vi "cam0#-搜索铜碎-2.vi"(8 "Cut基点":cluster{"X":sgl, "Y":sgl}, 9 "输入参数信息":T5, 11 "images":T4) -> (0 "存在铜碎":bool, 1 "检出点":cluster{"X":sgl, "Y":sgl}[](array[cluster]), 4 "ImageMorphOut":T1)   [LabVIEW 2018]
uses:
  <vilib>/vision/Image Controls.llb/IMAQ Image.ctl
  <vilib>/vision/NI_Vision_Development_Module.lvlib
panel:
  in  "槽口反光排除带区宽度":sgl=25.0
  out "ImageMorphOut 2":T1
  out "错误输出":errorcluster
  out "槽内存在铜碎异常":bool
  out "槽形态断裂情况":i32
  out "槽根部存在铜碎异常":bool
  in  "Keep/Remove Particles (F) 2":bool=TRUE
  in  "Selection Values 2":T3(array[cluster])=[{"Measurement Parameter"=35, "Range Lower Value"=0.0, "Range Upper Value"=50.0, "Range"=FALSE, "Measurement Type"=FALSE}] {"Measurement Parameter" items=["Center of Mass X", "Center of Mass Y", "First Pixel X", "First Pixel Y", "Bounding Rect Left", "Bounding Rect Top", "Bounding Rect Right", "Bounding Rect Bottom", "Max Feret Diameter Start X", "Max Feret Diameter Start Y", "Max Feret Diameter End X", "Max Feret Diameter End Y", "Max Horiz. Segment Length Left", "Max Horiz. Segment Length Right", "Max Horiz. Segment Length Row", "-", "Bounding Rect Width", "Bounding Rect Height", "Bounding Rect Diagonal", "Perimeter", "Convex Hull Perimeter", "Holes' Perimeter", "Max Feret Diameter", "Equivalent Ellipse Major Axis", "Equivalent Ellipse Minor Axis", "Equivalent Ellipse Minor Axis (Feret)", "Equivalent Rect Long Side", "Equivalent Rect Short Side", "Equivalent Rect Diagonal", "Equivalent Rect Short Side (Feret)", "Average Horiz. Segment Length", "Average Vert. Segment Length", "Hydraulic Radius", "Waddel Disk Diameter", "-", "Area", "Holes' Area", "Particle & Holes' Area", "Convex Hull Area", "Image Area", "-", "Number of Holes", "Number of Horiz. Segments", "Number of Vert. Segments", "-", "Orientation", "Max Feret Diameter Orientation", "-", "% Area/Image Area", "% Area/(Particle & Holes' Area)", "Ratio of Equivalent Ellipse Axes", "Ratio of Equivalent Rect Sides", "-", "Elongation Factor", "Compactness Factor", "Heywood Circularity Factor", "Type Factor", "-", "Sum X", "Sum Y", "Sum XX", "Sum XY", "Sum YY", "Sum XXX", "Sum XXY", "Sum XYY", "Sum YYY", "-", "Moment of Inertia XX", "Moment of Inertia XY", "Moment of Inertia YY", "Moment of Inertia XXX", "Moment of Inertia XXY", "Moment of Inertia XYY", "Moment of Inertia YYY", "Norm. Moment of Inertia XX", "Norm. Moment of Inertia XY", "Norm. Moment of Inertia YY", "Norm. Moment of Inertia XXX", "Norm. Moment of Inertia XXY", "Norm. Moment of Inertia XYY", "Norm. Moment of Inertia YYY", "Hu Moment 1", "Hu Moment 2", "Hu Moment 3", "Hu Moment 4", "Hu Moment 5", "Hu Moment 6", "Hu Moment 7"]; "Range Lower Value" format="%.2f"; "Range Upper Value" format="%.2f"}
  out "槽根部断裂型铜碎数量":i32
  in  "Keep/Remove Particles (F)":bool
  in  "Selection Values":T3(array[cluster])=[{"Measurement Parameter"=35, "Range Lower Value"=0.0, "Range Upper Value"=1000.0, "Range"=TRUE, "Measurement Type"=FALSE}] {"Measurement Parameter" items=["Center of Mass X", "Center of Mass Y", "First Pixel X", "First Pixel Y", "Bounding Rect Left", "Bounding Rect Top", "Bounding Rect Right", "Bounding Rect Bottom", "Max Feret Diameter Start X", "Max Feret Diameter Start Y", "Max Feret Diameter End X", "Max Feret Diameter End Y", "Max Horiz. Segment Length Left", "Max Horiz. Segment Length Right", "Max Horiz. Segment Length Row", "-", "Bounding Rect Width", "Bounding Rect Height", "Bounding Rect Diagonal", "Perimeter", "Convex Hull Perimeter", "Holes' Perimeter", "Max Feret Diameter", "Equivalent Ellipse Major Axis", "Equivalent Ellipse Minor Axis", "Equivalent Ellipse Minor Axis (Feret)", "Equivalent Rect Long Side", "Equivalent Rect Short Side", "Equivalent Rect Diagonal", "Equivalent Rect Short Side (Feret)", "Average Horiz. Segment Length", "Average Vert. Segment Length", "Hydraulic Radius", "Waddel Disk Diameter", "-", "Area", "Holes' Area", "Particle & Holes' Area", "Convex Hull Area", "Image Area", "-", "Number of Holes", "Number of Horiz. Segments", "Number of Vert. Segments", "-", "Orientation", "Max Feret Diameter Orientation", "-", "% Area/Image Area", "% Area/(Particle & Holes' Area)", "Ratio of Equivalent Ellipse Axes", "Ratio of Equivalent Rect Sides", "-", "Elongation Factor", "Compactness Factor", "Heywood Circularity Factor", "Type Factor", "-", "Sum X", "Sum Y", "Sum XX", "Sum XY", "Sum YY", "Sum XXX", "Sum XXY", "Sum XYY", "Sum YYY", "-", "Moment of Inertia XX", "Moment of Inertia XY", "Moment of Inertia YY", "Moment of Inertia XXX", "Moment of Inertia XXY", "Moment of Inertia XYY", "Moment of Inertia YYY", "Norm. Moment of Inertia XX", "Norm. Moment of Inertia XY", "Norm. Moment of Inertia YY", "Norm. Moment of Inertia XXX", "Norm. Moment of Inertia XXY", "Norm. Moment of Inertia XYY", "Norm. Moment of Inertia YYY", "Hu Moment 1", "Hu Moment 2", "Hu Moment 3", "Hu Moment 4", "Hu Moment 5", "Hu Moment 6", "Hu Moment 7"]}
  # "180110a-初始版本-测量槽宽"
  # "180126a-将基于边沿检测的铜碎搜索方法改为基于形态学的处理方法"
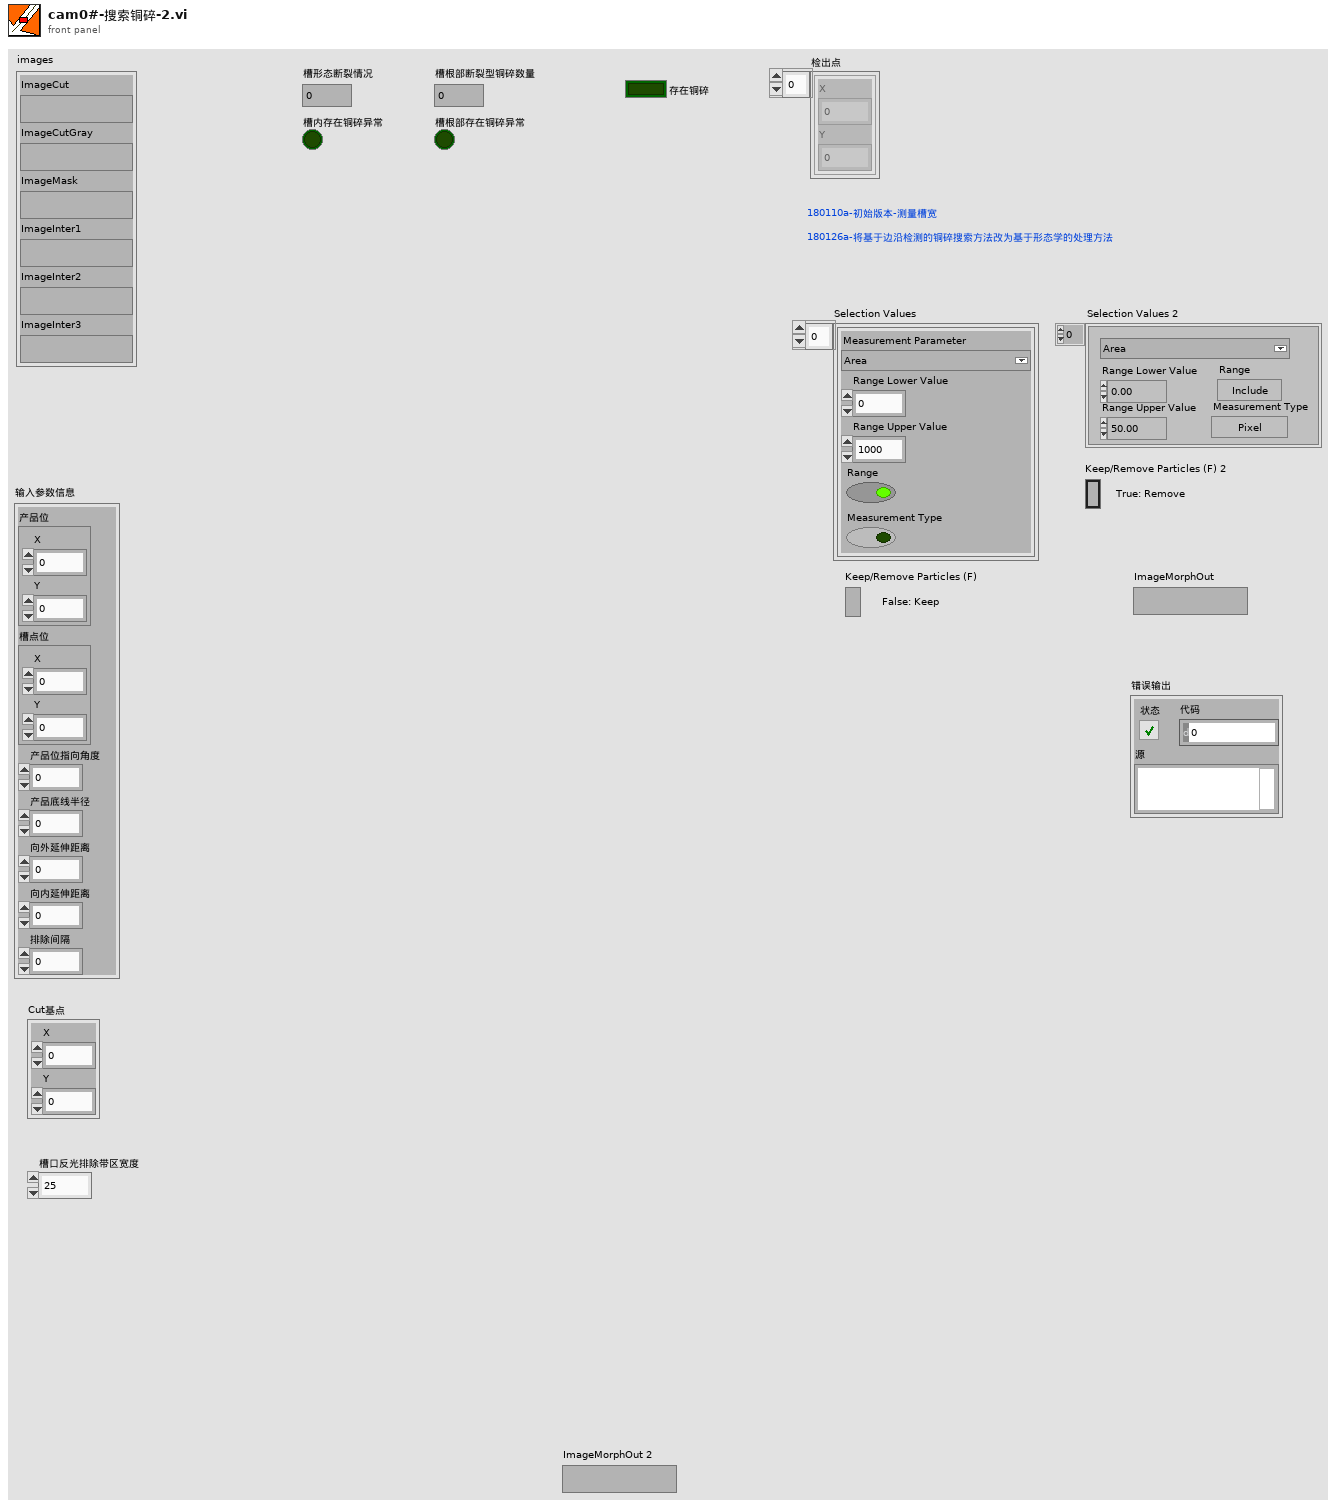
[diagram p1: front panel]
types:
  T1 = typedef "IMAQ Image.ctl" = refnum<image>
  T2 = typedef "Particle Parameters" = i32
  T3 = cluster{"Measurement Parameter":T2, "Range Lower Value":dbl, "Range Upper Value":dbl, "Range":bool, "Measurement Type":bool}[]
  T4 = cluster{"ImageCut":T1, "ImageCutGray":T1, "ImageMask":T1, "ImageInter1":T1, "ImageInter2":T1, "ImageInter3":T1}
  T5 = cluster{"产品位":cluster{"X":sgl, "Y":sgl}, "槽点位":cluster{"X":sgl, "Y":sgl}, "产品位指向角度":sgl, "产品底线半径":sgl, "向外延伸距离":sgl, "向内延伸距离":sgl, "排除间隔":sgl}
  T6 = typedef "IMAQ Circle" = cluster{"Center X":i32, "Center Y":i32, "Inner Radius":i32, "Outer Radius":i32, "Start Angle":dbl, "End Angle":dbl}
  T7 = enum32{"Average", "Min", "Max", "Clear  if < ", "Clear  if < or =", "Clear  if =", "Clear  if > or =", "Clear  if >"}
  T8 = enum32{"AutoM", "Close", "Dilate", "Erode", "Gradient", "Gradient out", "Gradient in", "Hit miss", "Open", "PClose", "POpen", "Thick", "Thin"}
  T9 = typedef "ROI Descriptor" = cluster{"Global Rectangle":i32[], "Contours":cluster{"ID":enum32{"External", "Internal"}, "Type":u32, "Coordinates":i32[]}[]}
  T10 = cluster{"Mean Intensity":sgl, "Standard  Deviation":sgl, "Minimum Intensity":sgl, "Maximum Intensity":sgl}
  T11 = cluster{"Starting Value":sgl, "Interval Width":sgl, "histogram":u32[]}
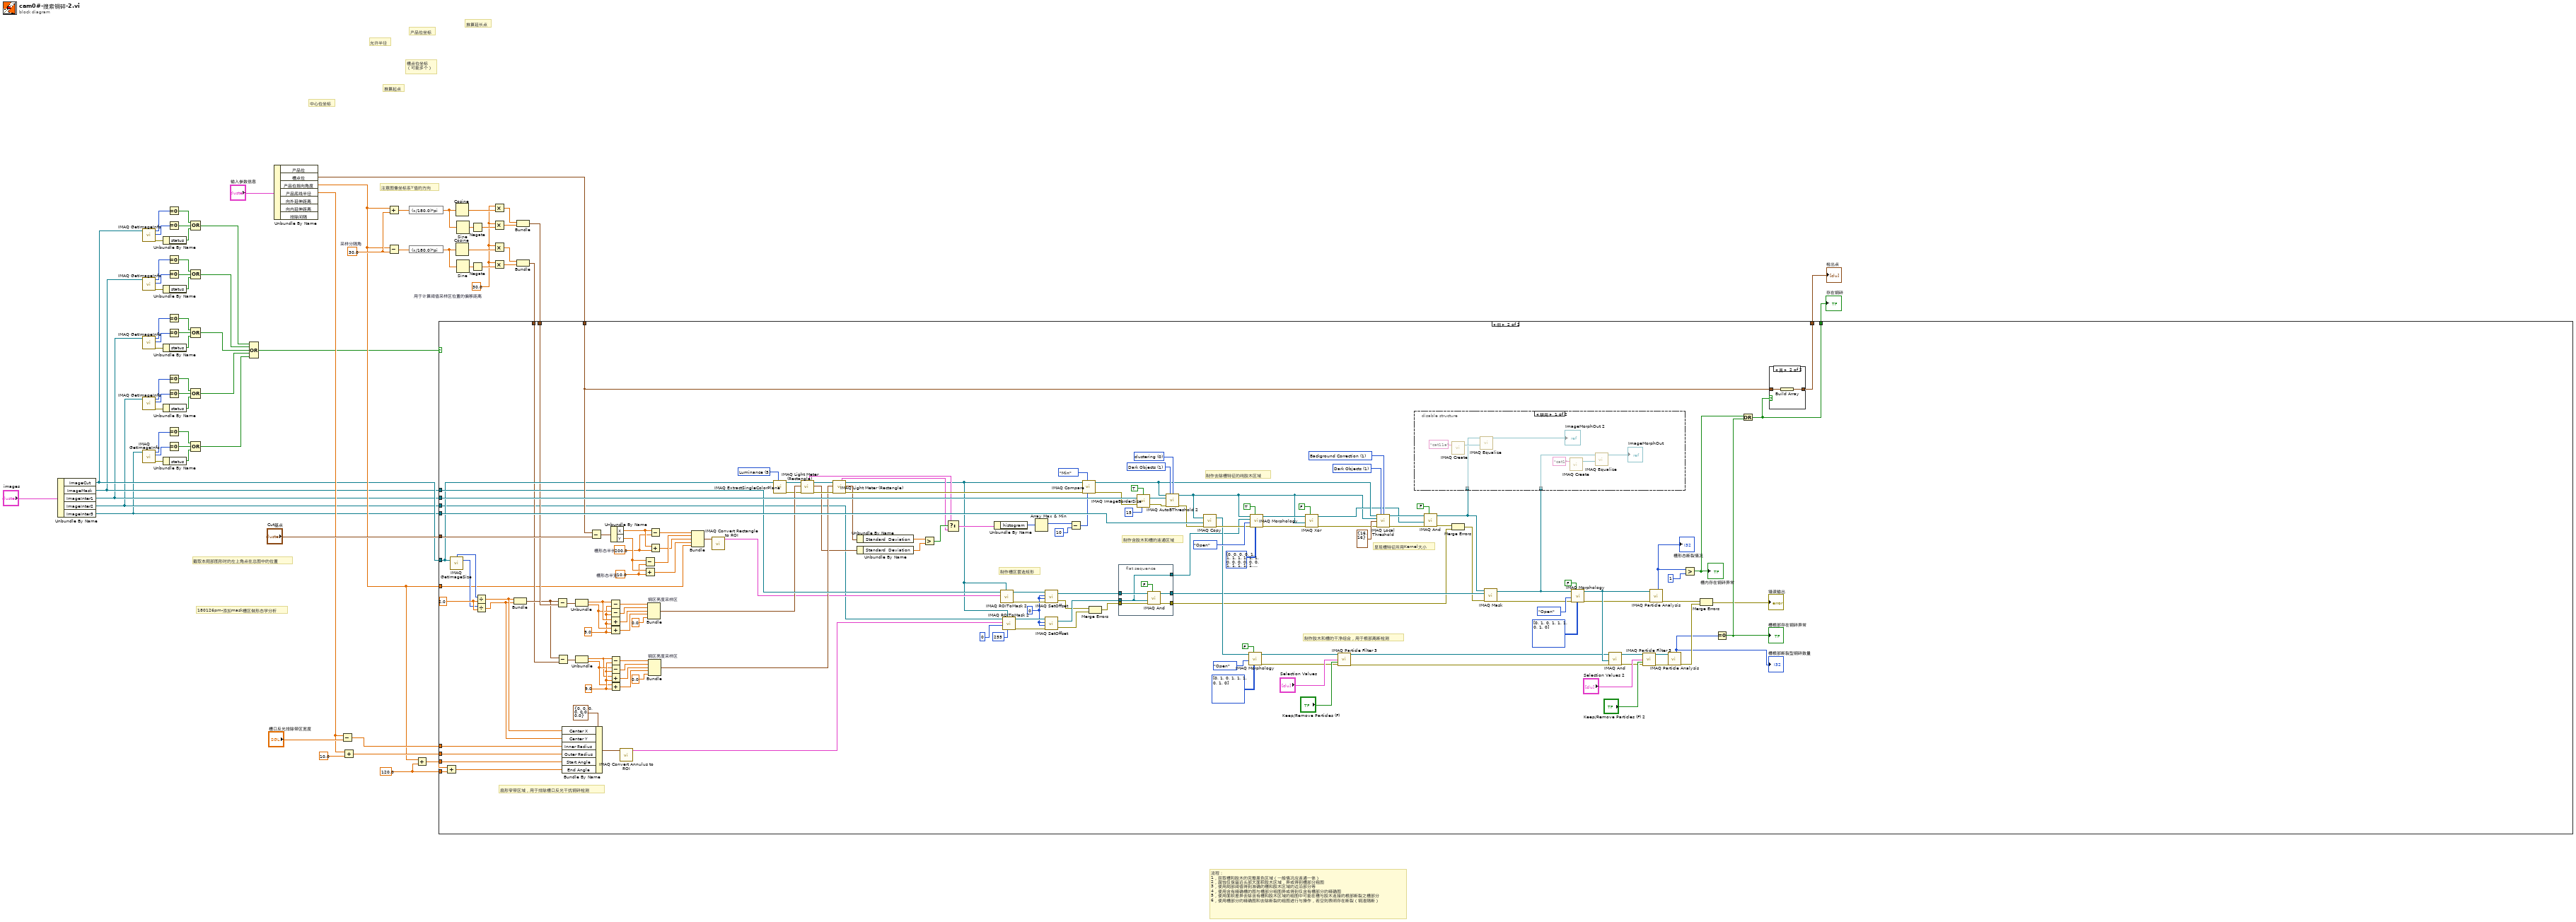
[diagram p0: block diagram]
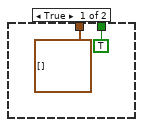
[diagram p2: hidden frame]
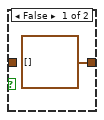
[diagram p4: hidden frame]
diagram:
  w47 = 120.0 ("y")
  w55 = sgl 30.0  # 采样分隔角
  w57 = sgl 30.0  # 用于计算阈值采样区位置的偏移距离
  # "截取本局部图形时的左上角点在总图中的位置"
  # "流程：\n1，获取槽和胶木的完整黑色区域（一般情况应连通一体）\n2，腐蚀仅保留近头部大面积胶木区域，异或得到槽部分粗图\n3，使用局部阈值得到准确的槽和胶木区域的边沿部分等\n4，使用含有精确槽的图与槽部分粗图异或得到仅含有槽部分的精确图\n5，使用面积差异去除含有槽和胶木区域的粗图中可能在槽与胶木连接的根部断裂之槽部分\n6，使用槽部分的精确图和去除断裂的粗图进行与操作，若空则表明存在断裂（铜渣隔断）"
  # "180126pm-添加mask槽区做形态学分析"
  # "注意图像坐标系Y值的方向"
  # "允许半径"
  # "推算起点"
  # "推算延长点"
  # "槽点位坐标\n（可能多个）"
  # "产品位坐标"
  # "中心位坐标"
  n1 = Unbundle By Name("images") -> ("ImageCut"=w13:T1, "ImageMask"=w12:T1, "ImageInter1"=w11:T1, "ImageInter2"=w10:T1, "ImageInter3"=w9:T1)
  n2 = call "IMAQ GetImageInfo"("Image"=w13) -> ("error out"=w17:errorcluster, "Y Resolution"=w18:i32, "X Resolution"=w19:i32)  [unwired: 3 in, 5 out]
  n3 = call "IMAQ GetImageInfo"("Image"=w12) -> ("error out"=w22:errorcluster, "Y Resolution"=w21:i32, "X Resolution"=w20:i32)  [unwired: 3 in, 5 out]
  n4 = call "IMAQ GetImageInfo"("Image"=w11) -> ("error out"=w29:errorcluster, "Y Resolution"=w30:i32, "X Resolution"=w31:i32)  [unwired: 3 in, 5 out]
  n5 = call "IMAQ GetImageInfo"("Image"=w10) -> ("error out"=w41:errorcluster, "Y Resolution"=w42:i32, "X Resolution"=w43:i32)  [unwired: 3 in, 5 out]
  n6 = call "IMAQ GetImageInfo"("Image"=w9) -> ("error out"=w34:errorcluster, "Y Resolution"=w33:i32, "X Resolution"=w32:i32)  [unwired: 3 in, 5 out]
  n7 = Unbundle By Name(w17) -> ("status"=w14:bool)
  n8 = Unbundle By Name(w22) -> ("status"=w25:bool)
  n9 = Unbundle By Name(w29) -> ("status"=w26:bool)
  n10 = Unbundle By Name(w41) -> ("status"=w38:bool)
  n11 = Unbundle By Name(w34) -> ("status"=w37:bool)
  n12 = Equal To 0?(x=w19) -> (x = 0?=w16:bool)
  n13 = Equal To 0?(x=w18) -> (x = 0?=w15:bool)
  n14 = Equal To 0?(x=w20) -> (x = 0?=w23:bool)
  n15 = Equal To 0?(x=w21) -> (x = 0?=w24:bool)
  n16 = Equal To 0?(x=w31) -> (x = 0?=w28:bool)
  n17 = Equal To 0?(x=w30) -> (x = 0?=w27:bool)
  n18 = Equal To 0?(x=w43) -> (x = 0?=w40:bool)
  n19 = Equal To 0?(x=w42) -> (x = 0?=w39:bool)
  n20 = Equal To 0?(x=w32) -> (x = 0?=w35:bool)
  n21 = Equal To 0?(x=w33) -> (x = 0?=w36:bool)
  n22 = Compound Arithmetic op=OR ("复合运算")(w16, w15, w14) -> (w8:bool)
  n23 = Compound Arithmetic op=OR ("复合运算")(w23, w24, w25) -> (w7:bool)
  n24 = Compound Arithmetic op=OR ("复合运算")(w28, w27, w26) -> (w6:bool)
  n25 = Compound Arithmetic op=OR ("复合运算")(w40, w39, w38) -> (w5:bool)
  n26 = Compound Arithmetic op=OR ("复合运算")(w35, w36, w37) -> (w4:bool)
  n27 = Compound Arithmetic op=OR ("复合运算")(w8, w7, w6, w5, w4) -> (w3:bool)
  n28 = Unbundle By Name("输入参数信息") -> ("槽点位"=w69:cluster{"X":sgl, "Y":sgl}, "产品位指向角度"=w46:sgl, "产品底线半径"=w50:sgl)  [unwired: 4 out]
  n29 = Subtract(x=w50, y="槽口反光排除带区宽度") -> (x-y=w51:sgl)
  n30 = Add(x=w50, y=sgl 10.0) -> (x+y=w48:sgl)
  n31 = Add(x=w46, y=w55) -> (x+y=w64:sgl)
  n32 = Subtract(x=w46, y=w55) -> (x-y=w56:sgl)
  n33 = expression code="(x/180.0)*pi" ("degrees to radians")(w64) -> (w73:sgl)
  n34 = expression code="(x/180.0)*pi" ("degrees to radians")(w56) -> (w58:sgl)
  n35 = Add(x=w46, y=w47) -> (x+y=w45:dbl)
  n36 = Cosine(x=w73) -> (cos(x)=w66:sgl)
  n37 = Cosine(x=w58) -> (cos(x)=w62:sgl)
  n38 = Sine(x=w73) -> (sin(x)=w71:sgl)
  n39 = Sine(x=w58) -> (sin(x)=w59:sgl)
  n40 = Negate(x=w71) -> (-x=w65:sgl)
  n41 = Negate(x=w59) -> (-x=w63:sgl)
  n42 = Multiply(x=w57, y=w66) -> (x*y=w68:sgl)
  n43 = Multiply(x=w57, y=w65) -> (x*y=w67:sgl)
  n44 = Multiply(x=w57, y=w62) -> (x*y=w60:sgl)
  n45 = Multiply(x=w57, y=w63) -> (x*y=w61:sgl)
  n46 = Bundle(w68, w67) -> (w54:cluster{sgl, sgl})  [unwired: 1 in]
  n47 = Bundle(w60, w61) -> (w53:cluster{sgl, sgl})  [unwired: 1 in]
  n48 = case shown="假" w3 {
    tunnel: "Cut基点" -> [_ w219]
    tunnel: w11 -> [_ w200]
    tunnel: w9 -> [_ w197]
    tunnel: w69 -> [_ w176]
    tunnel: w12 -> [_ w175]
    tunnel: w13 -> [_ w162]
    tunnel: w54 -> [_ w140]
    tunnel: w53 -> [_ w138]
    tunnel: w51 -> [_ w114]
    tunnel: w48 -> [_ w113]
    tunnel: w47 -> [_ w112]
    tunnel: w46 -> [_ w111]
    tunnel: w45 -> [_ w108]
    tunnel: w10 -> [_ w83]
    tunnel: [cluster{"X":sgl, "Y":sgl}[] [] w77] -> w2
    tunnel: [TRUE w76] -> w1
    frame True {
    }
    frame False {
      w93 = 0 ("X Offset")
      w144 = sgl 9.0 ("y")
      w165 = 2.0 ("y")
      w171 = sgl 9.0 ("y")
      w205 = u32 1 items=["Bright Objects", "Dark Objects"] ("Look For (Bright Objects)")
      w207 = u32 1 items=["Niblack", "Background Correction"] ("Method")
      w211 = 0 items=["clustering", "entropy", "metric", "moments", "inter-class variance"] ("Method")
      w212 = u32 1 items=["Bright Objects", "Dark Objects"] ("Look For")
      w213 = 5 items=["Red", "Green", "Blue", "Hue", "Saturation", "Luminance", "Value", "Intensity"] ("Color Plane")
      w214 = sgl 200.0  # 槽形态半长
      w224 = sgl 10.0  # 槽形态半宽
      # "扇形窄带区域，用于排除槽口反光干扰铜碎检测"
      # "显现槽特征所用Kernel大小"
      # "制作去除槽特征的纯胶木区域"
      # "制作含胶木和槽的连通区域"
      # "制作胶木和槽的干净组合，用于根部离断检测"
      # "制作槽区套选矩形"
      n49 = Add(x=w108, y=w112) -> (x+y=w110:dbl)
      n50 = call "IMAQ GetImageSize"("Image"=w162) -> ("Y Resolution"=w163:i32, "X Resolution"=w164:i32)  [unwired: 3 in, 1 out]
      n51 = Divide(x=w164, y=w165) -> (x/y=w116:dbl)
      n52 = Divide(x=w163, y=w165) -> (x/y=w115:dbl)
      n53 = Bundle(w116, w115) -> (w139:cluster{dbl, dbl})  [unwired: 1 in]
      n54 = Subtract(x=w139, y=w140) -> (x-y=w174:cluster{dbl, dbl})
      n55 = Subtract(x=w139, y=w138) -> (x-y=w141:cluster{dbl, dbl})
      n56 = Bundle By Name(cluster=T6 {"Center X"=0, "Center Y"=0, "Inner Radius"=0, "Outer Radius"=0, "Start Angle"=0.0, "End Angle"=0.0} ("Annulus"), "Center X"=w116, "Center Y"=w115, "Inner Radius"=w114, "Outer Radius"=w113, "Start Angle"=w108, "End Angle"=w110) -> (w117:T6)
      n57 = Unbundle(w174) -> (w173:dbl, w172:dbl)
      n58 = Unbundle(w141) -> (w142:dbl, w143:dbl)
      n59 = Subtract(x=w176, y=w219) -> (x-y=w215:cluster{"X":sgl, "Y":sgl})
      n60 = Subtract(x=w173, y=w171) -> (x-y=w170:dbl)
      n61 = Subtract(x=w172, y=w171) -> (x-y=w169:dbl)
      n62 = Add(x=w173, y=w171) -> (x+y=w168:dbl)
      n63 = Add(x=w172, y=w171) -> (x+y=w167:dbl)
      n64 = Subtract(x=w142, y=w144) -> (x-y=w145:dbl)
      n65 = Subtract(x=w143, y=w144) -> (x-y=w146:dbl)
      n66 = Add(x=w142, y=w144) -> (x+y=w147:dbl)
      n67 = Add(x=w143, y=w144) -> (x+y=w148:dbl)
      n68 = Unbundle By Name(w215) -> ("X"=w226:sgl, "Y"=w225:sgl)
      n69 = call "IMAQ Convert Annulus to ROI"("Annulus"=w117) -> ("ROI Descriptor"=w106:T9)  [unwired: 8 in, 1 out]
      n70 = Subtract(x=w225, y=w224) -> (x-y=w222:sgl)
      n71 = Add(x=w225, y=w224) -> (x+y=w220:sgl)
      n72 = Bundle "铜区亮度采样区"(w170, w169, w168, w167, "y"=sgl 0.0) -> (w160:cluster{dbl, dbl, dbl, dbl, "y":sgl})  [unwired: 1 in]
      n73 = Bundle "铜区亮度采样区"(w145, w146, w147, w148, "y"=sgl 0.0) -> (w134:cluster{dbl, dbl, dbl, dbl, "y":sgl})  [unwired: 1 in]
      n74 = Subtract(x=w226, y=w214) -> (x-y=w223:sgl)
      n75 = Add(x=w226, y=w214) -> (x+y=w221:sgl)
      n76 = Bundle(w223, w222, w221, w220, "产品位指向角度"=w111) -> (w218:cluster{sgl, sgl, sgl, sgl, "产品位指向角度":sgl})  [unwired: 1 in]
      n77 = call "IMAQ Convert Rectangle to ROI"("Rectangle"=w218) -> ("ROI Descriptor"=w109:T9)  [unwired: 8 in, 1 out]
      n78 = call "IMAQ ExtractSingleColorPlane"("Color Plane"=w213, "Image Src"=w162) -> ("error out"=w150:errorcluster, "Image Dst Out"=w154:T1)  [unwired: 8 in]
      n79 = call "IMAQ Light Meter (Rectangle)"("error in (no error)"=w150, "Rectangle"=w160, "Image"=w154) -> ("error out"=w136:errorcluster, "Gray Level Intensities"=w132:T10, "Image Out"=w137:T1, "Histogram"=w128:T11)  [unwired: 4 in, 1 out]
      n80 = call "IMAQ Light Meter (Rectangle)"("error in (no error)"=w136, "Rectangle"=w134, "Image"=w137) -> ("error out"=w135:errorcluster, "Gray Level Intensities"=w133:T10, "Image Out"=w81:T1, "Histogram"=w127:T11)  [unwired: 4 in, 1 out]
      n81 = Unbundle By Name(w133) -> ("Standard  Deviation"=w131:sgl)
      n82 = Unbundle By Name(w132) -> ("Standard  Deviation"=w130:sgl)
      n83 = Greater?(x=w131, y=w130) -> (0:w129:bool)
      n84 = Select(t=w128, s=w129, f=w127) -> (s? t:f=w126:T11)
      n85 = Unbundle By Name(w126) -> ("histogram"=w158:u32[])
      n86 = call "IMAQ ROIToMask 2"("Image Model"=w81, "ROI Descriptor"=w109, "Image"=w175) -> ("error out"=w216:errorcluster, "Image Out"=w217:T1)  [unwired: 6 in, 1 out]
      n87 = call "IMAQ ROIToMask 2"("Background Value (0)"=255, "Image Model"=w81, "Filling Value (255)"=0, "ROI Descriptor"=w106, "Image"=w83) -> ("error out"=w107:errorcluster, "Image Out"=w105:T1)  [unwired: 4 in, 1 out]
      n88 = Array Max & Min(array=w158) -> (max index (indices)=w155:i32)  [unwired: 3 out]
      n89 = call "IMAQ SetOffset"("error in (no error)"=w216, "Y Offset"=w93, "X Offset"=w93, "Image"=w217) -> ("error out"=w87:errorcluster, "Image Out"=w89:T1)
      n90 = call "IMAQ SetOffset"("error in (no error)"=w107, "Y Offset"=w93, "X Offset"=w93, "Image"=w105) -> ("error out"=w86:errorcluster, "Image Out"=w91:T1)
      n91 = Subtract(x=w155, y=u32 10) -> (x-y=w156:u32)
      n92 = call "IMAQ Compare"("Constant"=w156, "Operator"=T7."Min", "error in (no error)"=w135, "Image Src A"=w81) -> ("error out"=w159:errorcluster, "Image Dst Out"=w119:T1)  [unwired: 6 in]
      n93 = Merge Errors(w87, w86) -> (w85:errorcluster)
      n94 = flat-sequence {
        tunnel: w91 -> [w235]
        tunnel: w89 -> [w239]
        tunnel: [w238] -> w88
        tunnel: w85 -> [w237]
        tunnel: [w236] -> w84
        tunnel: [w235] -> w82
        frame #0 {
          n95 = call "IMAQ And"("And/Nand (And)"=FALSE, "error in (no error)"=w237, "Image Src B"=w235, "Image Src A"=w239) -> ("error out"=w236:errorcluster, "Image Dst Out"=w238:T1)  [unwired: 2 in, 4 out]
        }
      }
      n96 = call "IMAQ ImageBorderSize"("Get/Set Status? (Set)"=TRUE, "Image"=w200, "Image border size in"=15 ("Border Size"), "error in (no error)"=w159) -> ("Image Out"=w199:T1, "error out"=w201:errorcluster)  [unwired: 1 out]
      n97 = call "IMAQ AutoBThreshold 2"("Image Src"=w119, "Look For (Bright Objects)"=w212, "Method (clustering)"=w211, "Image Dst"=w199, "error in (no error)"=w201) -> ("Image Dst Out"=w99:T1, "error out"=w80:errorcluster)  [unwired: 3 in, 6 out]
      n98 = call "IMAQ Copy"("error in (no error)"=w80, "Image Dst"=w197, "Image Src"=w99) -> ("error out"=w198:errorcluster, "Image Dst Out"=w121:T1)  [unwired: 3 in]
      n99 = call "IMAQ Morphology"("Structuring Element"=i32[][] [[0, 1, 0], [1, 1, 1], [0, 1, 0]], "Square/Hexa (Square)"=FALSE, "Operation"=T8."Open", "Image Src"=w121) -> ("error out"=w191:errorcluster, "Image Dst Out"=w122:T1)  [unwired: 6 in]
      n100 = call "IMAQ Morphology"("Structuring Element"=i32[][] [[0, 0, 0, 0, 1, 1, 1, 1, 1, 1, 1, 0, 0, 0, 0], [0, 0, 1, 1, 1, 1, 1, 1, 1, 1, 1, 1, 1, 0, 0], [0, 1, 1, 1, 1, 1, 1, 1, 1, 1, 1, 1, 1, 1, 0], [0, 1, 1, 1, 1, 1, 1, 1, 1, 1, 1, 1, 1, 1, 0], [1, 1, 1, 1, 1, 1, 1, 1, 1, 1, 1, 1, 1, 1, 1], [1, 1, 1, 1, 1, 1, 1, 1, 1, 1, 1, 1, 1, 1, 1], [1, 1, 1, 1, 1, 1, 1, 1, 1, 1, 1, 1, 1, 1, 1], [1, 1, 1, 1, 1, 1, 1, 1, 1, 1, 1, 1, 1, 1, 1], [1, 1, 1, 1, 1, 1, 1, 1, 1, 1, 1, 1, 1, 1, 1], [1, 1, 1, 1, 1, 1, 1, 1, 1, 1, 1, 1, 1, 1, 1], [1, 1, 1, 1, 1, 1, 1, 1, 1, 1, 1, 1, 1, 1, 1], [0, 1, 1, 1, 1, 1, 1, 1, 1, 1, 1, 1, 1, 1, 0], [0, 1, 1, 1, 1, 1, 1, 1, 1, 1, 1, 1, 1, 1, 0], [0, 0, 1, 1, 1, 1, 1, 1, 1, 1, 1, 1, 1, 0, 0], [0, 0, 0, 0, 1, 1, 1, 1, 1, 1, 1, 0, 0, 0, 0]] ("Structuring Element (Basic Morphology 2)"), "Square/Hexa (Square)"=TRUE, "error in (no error)"=w198, "Operation"=T8."Open", "Image Dst"=w82, "Image Src"=w99) -> ("error out"=w92:errorcluster, "Image Dst Out"=w100:T1)  [unwired: 1 in, 3 out]
      n101 = call "IMAQ Xor"("Xor/Xnor (Xor)"=FALSE, "error in (no error)"=w92, "Image Src B"=w99, "Image Src A"=w100) -> ("error out"=w101:errorcluster, "Image Dst Out"=w102:T1)  [unwired: 2 in, 4 out]
      n102 = call "IMAQ Particle Filter 3"("Image Src"=w122, "Selection Values"="Selection Values", "Keep/Remove Particles (F)"="Keep/Remove Particles (F)", "error in (no error)"=w191) -> ("Image Dst Out"=w123:T1, "error out"=w124:errorcluster)  [unwired: 9 in, 1 out]
      n103 = call "IMAQ Local Threshold"("Image Src"=w119, "Look For (Bright Objects)"=w205, "Method (Niblack)"=w207, "Image Dst"=w99, "Window Size (32x32)"=cluster{"SizeX":i32, "SizeY":i32} {"SizeX"=16, "SizeY"=16} ("Kernel Size"), "error in (no error)"=w101) -> ("Image Dst Out"=w103:T1, "error out"=w97:errorcluster)  [unwired: 3 in, 5 out]
      n104 = call "IMAQ And"("And/Nand (And)"=FALSE, "error in (no error)"=w97, "Image Src B"=w102, "Image Src A"=w103) -> ("error out"=w125:errorcluster, "Image Dst Out"=w96:T1)  [unwired: 2 in, 4 out]
      n105 = Merge Errors(w125, w84) -> (w79:errorcluster)
      n106 = call "IMAQ Mask"("error in (no error)"=w79, "Image Mask"=w88, "Image Src"=w96) -> ("error out"=w78:errorcluster, "Image Dst Out"=w90:T1)  [unwired: 2 in]
      n107 = disable-structure shown="禁用" {
        disable-tunnel: w96 -> [w228 _]
        disable-tunnel: w90 -> [w227 _]
        frame Disabled {
          n108 = call "IMAQ Create"("Image Name"="cat11a") -> ("New Image"=w231:T1)  [unwired: 4 in, 1 out]
          n109 = call "IMAQ Equalize"("Image Dst"=w231, "Image Src"=w228) -> ("Image Dst Out"=→"ImageMorphOut 2":T1)  [unwired: 8 in, 1 out]
          n110 = call "IMAQ Create"("Image Name"="cat1") -> ("New Image"=w232:T1)  [unwired: 4 in, 1 out]
          n111 = call "IMAQ Equalize"("Image Dst"=w232, "Image Src"=w227) -> ("Image Dst Out"=→"ImageMorphOut":T1)  [unwired: 8 in, 1 out]
        }
        frame Enabled {
        }
      }
      n112 = call "IMAQ Morphology"("Structuring Element"=i32[][] [[0, 1, 0], [1, 1, 1], [0, 1, 0]], "Square/Hexa (Square)"=FALSE, "error in (no error)"=w78, "Operation"=T8."Open", "Image Src"=w90) -> ("error out"=w95:errorcluster, "Image Dst Out"=w152:T1)  [unwired: 5 in]
      n113 = call "IMAQ And"("error in (no error)"=w124, "Image Src B"=w152, "Image Src A"=w123) -> ("error out"=w185:errorcluster, "Image Dst Out"=w120:T1)  [unwired: 3 in, 4 out]
      n114 = call "IMAQ Particle Filter 3"("Image Src"=w120, "Selection Values"="Selection Values 2", "Keep/Remove Particles (F)"="Keep/Remove Particles (F) 2", "error in (no error)"=w185) -> ("Image Dst Out"=w186:T1, "error out"=w189:errorcluster)  [unwired: 9 in, 1 out]
      n115 = call "IMAQ Particle Analysis"("error in (no error)"=w95, "Image"=w152) -> ("error out"=w181:errorcluster, "Number of Particles"=w180:i32)  [unwired: 4 in, 4 out]
      "槽形态断裂情况" <- w180
      n116 = call "IMAQ Particle Analysis"("error in (no error)"=w189, "Image"=w186) -> ("error out"=w190:errorcluster, "Number of Particles"=w153:i32)  [unwired: 4 in, 4 out]
      "槽根部断裂型铜碎数量" <- w153
      n117 = Greater?(x=w180, y=1) -> (0:w178:bool)
      "槽内存在铜碎异常" <- w178
      n118 = Merge Errors(w181, w190) -> (→"错误输出":errorcluster)
      n119 = Equal To 0?(x=w153) -> (x = 0?=w177:bool)
      "槽根部存在铜碎异常" <- w177
      n120 = Or(x=w178, y=w177) -> (x .or. y?=w76:bool)
      n121 = case shown="真" w76 {
        tunnel: w176 -> [_ w243]
        tunnel: [cluster{"X":sgl, "Y":sgl}[] [] w242] -> w77
        frame False {
        }
        frame True {
          n122 = Build Array(w243) -> (w242:cluster{"X":sgl, "Y":sgl}[])
        }
      }
    }
  }
  "存在铜碎" <- w1
  "检出点" <- w2
